vi "local drive robot.vi"() -> ()   [LabVIEW 2018]
uses:
  <vilib>/MakerHub/Xbox-One-Controller/Public/Open First Controller.vi
  <vilib>/MakerHub/Xbox-One-Controller/LMH-Xbox-One-Controller.lvlib
panel:
  in  "milliseconds to wait":u32=10
  in  "Reverse y-axis?":bool=TRUE
  in  "Reverse x-axis?":bool=TRUE
  in  "Deadband value (0)":i32
  in  "Max controller reading":dbl=29767.0
  in  "deadband limit":i32=3000
  in  "stop":bool
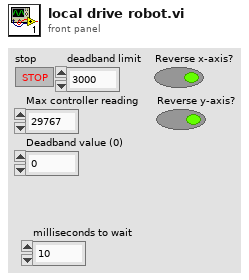
[diagram p1: front panel]
types:
  T1 = typedef "LMH-Xbox-One-Controller.lvlib/Xbox One Controller Ref.ctl" = cluster{"Controller Ref":refnum<k1>, "Event Refnum":refnum<event-registration>, "Worker Ref":refnum<vi>}
  T2 = typedef "LMH-Xbox-One-Controller.lvlib/All Axis Data.ctl" = cluster{"Left Stick":cluster{"X Axis":i32, "Y Axis":i32}, "Right Stick":cluster{"X Axis":i32, "Y Axis":i32}, "Triggers":i32, "D-Pad":T3}
  T3 = typedef "LMH-Xbox-One-Controller.lvlib/DPad Enum.ctl" = enum16{"Idle", "Up", "Up / Right", "Right", "Down / Right", "Down", "Down / Left", "Left", "Up / Left"}
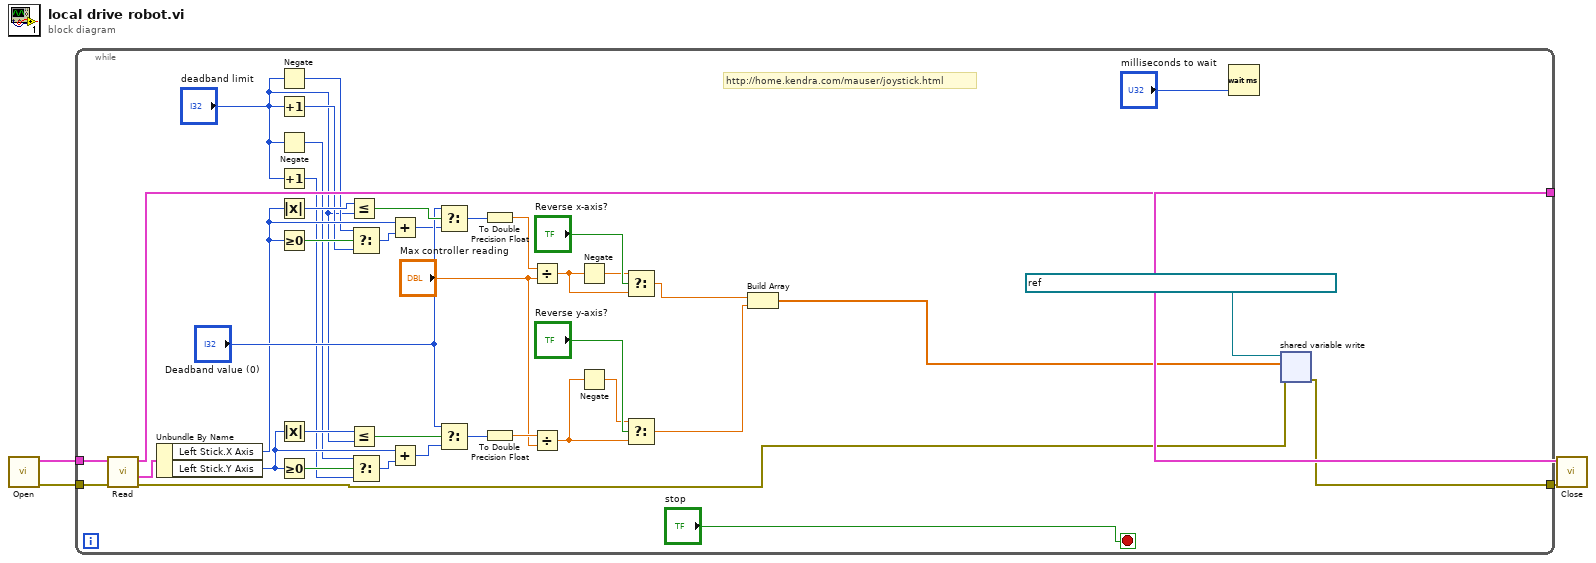
[diagram p0: block diagram]
diagram:
  n1 = call-poly <vilib>:"Open.vi"() -> ("Error Out"=w2:errorcluster, "Xbox One Controller"=w4:T1)  [unwired: 9 in, 1 out]
  n2 = while {
    tunnel: w2 -> [w43]
    tunnel: [w10] -> w1
    tunnel: w4 -> [w45]
    tunnel: [w44] -> w3
    stop <- "stop" stop-if-true
    # "http://home.kendra.com/mauser/joystick.html"
    n3 = call <vilib>:"Read.vi"("Error In"=w43, "Xbox One Controller Ref"=w45) -> ("Error Out"=w11:errorcluster, "All Axis"=w42:T2, "Xbox One Controller Ref"=w44:T1)  [unwired: 6 in, 1 out]
    n4 = Unbundle By Name(w42) -> ("Left Stick.X Axis"=w32:i32, "Left Stick.Y Axis"=w28:i32)
    n5 = Negate(x="deadband limit") -> (-x=w22:i32)
    n6 = Increment(x="deadband limit") -> (x+1=w21:i32)
    n7 = Negate(x="deadband limit") -> (-x=w20:i32)
    n8 = Increment(x="deadband limit") -> (x+1=w19:i32)
    n9 = Absolute Value(x=w32) -> (abs(x)=w37:i32)
    n10 = Greater Or Equal To 0?(x=w32) -> (x >= 0?=w33:bool)
    n11 = Absolute Value(x=w28) -> (abs(x)=w36:i32)
    n12 = Greater Or Equal To 0?(x=w28) -> (x >= 0?=w30:bool)
    n13 = Less Or Equal?(x=w37, y="deadband limit") -> (x <= y?=w39:bool)
    n14 = Less Or Equal?(x=w36, y="deadband limit") -> (x <= y?=w40:bool)
    n15 = Select(t=w22, s=w33, f=w21) -> (s? t:f=w31:i32)
    n16 = Select(t=w20, s=w30, f=w19) -> (s? t:f=w29:i32)
    n17 = Add(x=w32, y=w31) -> (x+y=w35:i32)
    n18 = Add(x=w28, y=w29) -> (x+y=w34:i32)
    n19 = Select(t="Deadband value (0)", s=w39, f=w35) -> (s? t:f=w27:i32)
    n20 = Select(t="Deadband value (0)", s=w40, f=w34) -> (s? t:f=w26:i32)
    n21 = To Double Precision Float(number=w27) -> (double precision float=w25:dbl)
    n22 = To Double Precision Float(number=w26) -> (double precision float=w24:dbl)
    n23 = Divide(x=w25, y="Max controller reading") -> (x/y=w15:dbl)
    n24 = Divide(x=w24, y="Max controller reading") -> (x/y=w13:dbl)
    n25 = Negate(x=w15) -> (-x=w14:dbl)
    n26 = Negate(x=w13) -> (-x=w12:dbl)
    n27 = Select(t=w14, s="Reverse x-axis?", f=w15) -> (s? t:f=w8:dbl)
    n28 = Select(t=w12, s="Reverse y-axis?", f=w13) -> (s? t:f=w7:dbl)
    n29 = Build Array(w8, w7) -> (w6:dbl[])
    n30 = Wait (ms)(milliseconds to wait="milliseconds to wait") -> ()  [unwired: 1 out]
    n31 = shared-variable-write(refnum<k21> "ni.var.psp://karims-myrio/Motor Speeds/CTL X %26 Y" ("shared variable refnum in"), w11, w6) -> (w10:errorcluster)  [unwired: 1 out]
  }
  n32 = call <vilib>:"Close.vi"("Error In"=w1, "Xbox One Controller Ref"=w3) -> ()  [unwired: 9 in, 1 out]
